vi "SaveGestureType.vi"(11 "Type":i32(ring)=-1 items=["TYPESWIPE"=1, "TYPECIRCLE"=4, "TYPESCREENTAP"=5, "TYPEKEYTAP"=6, "TYPEINVALID"=-1]) -> (3 "gesture type":T1)   [LabVIEW 2010, in "lvleap.lvlib"]
uses:
  lvleap.lvlib
  Controls/Gesture Type.ctl
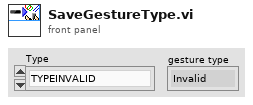
[diagram p1: front panel]
types:
  T1 = typedef "lvleap.lvlib/Gesture Type.ctl" = enum16{"Invalid", "Swipe", "Circle", "Screen Tap", "Key Tap"}
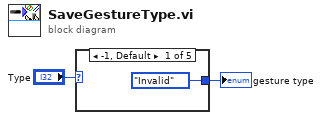
[diagram p0: block diagram]
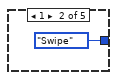
[diagram p2: hidden frame]
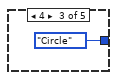
[diagram p3: hidden frame]
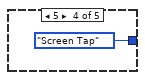
[diagram p4: hidden frame]
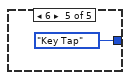
[diagram p5: hidden frame]
diagram:
  n1 = case shown="-1, Default" "Type" {
    tunnel: [Gesture_Type."Invalid" ("gesture type") Gesture_Type."Swipe" ("gesture type") Gesture_Type."Circle" ("gesture type") Gesture_Type."Screen Tap" ("gesture type") Gesture_Type."Key Tap" ("gesture type")] -> w1
    frame -1, Default {
    }
    frame 1 {
    }
    frame 4 {
    }
    frame 5 {
    }
    frame 6 {
    }
  }
  "gesture type" <- w1
